vi "SetClassQueue.vi"(8 "ErrorIn(No Error)":errorcluster caption="entrée d'erreur (pas d'erreur)", 11 "PhotoLum.lvclass":refnum<class "PhotoLum.lvclass">) -> (0 "sortie d'erreur":errorcluster, 3 "PhotoLum.lvclass Out":refnum<class "PhotoLum.lvclass">)   [LabVIEW 2010, in "PhotoLum.lvclass"]
uses:
  PhotoLum.lvclass
  BaseDevice/BaseDevice.lvclass
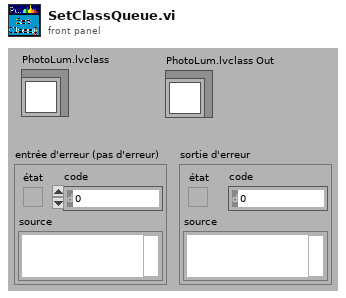
[diagram p1: front panel]
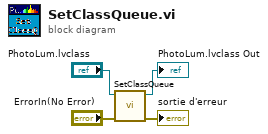
[diagram p0: block diagram]
diagram:
  n1 = call-parent "SetClassQueue.vi"("ErrorIn(No Error)"="ErrorIn(No Error)", "BaseDevice.lvclass"="PhotoLum.lvclass") -> ("sortie d'erreur"=→"sortie d'erreur":errorcluster, "BaseDevice.lvclass Out"=→"PhotoLum.lvclass Out":refnum<class "PhotoLum.lvclass">)  [unwired: 8 in]
